vi "Teleop.vi"(10 "Match Info":T1={"Autonomous Elapsed Seconds"=0.0, "TeleOp Elapsed Seconds"=0.0, "Disabled Elapsed Seconds"=0.0, "Visited Autonomous"=FALSE, "Visited TeleOp"=FALSE, "Visited Disabled"=FALSE, "Autonomous Settings"={"Autonomous Style"=enum."Independent", "VI Refnum"=refnum}}, 11 "Call Context":T2) -> ()   [LabVIEW 2019]
doc: "This VI is called for each TeleOp packet received from the DS where the robot is not disabled. It is often used to read from the joysticks and update I/O or to update setpoints for timed control loops. It should complete and return within 20 milliseconds or it may miss DS packets."
uses:
  <vilib>/Rock Robotics/WPI/DriverStation/WPI_DriverStationDerivedRobotMode.ctl
  <vilib>/Rock Robotics/WPI/DriverStation/WPI_DriverStationMatch Info.ctl
  <vilib>/Rock Robotics/WPI/ThirdParty/JAS_Junk/TrajLib/Conv_Meters_Feet.vi
  <vilib>/Rock Robotics/WPI/ThirdParty/JAS_Junk/TrajLib/Conv_Radians_Deg.vi
  <vilib>/Rock Robotics/WPI/Utilities/WPI_GetSetVariantRefNum.vi
  <vilib>/Rock Robotics/Network Tables/NT Write Boolean Array.vi
  <vilib>/Rock Robotics/Network Tables/NT Write Numeric Array.vi
  <vilib>/Rock Robotics/WPI/Joystick/WPI_JoystickArcadeMapping.vi
  Robot Global Data.vi
  <vilib>/Rock Robotics/Network Tables/NT Read Boolean.vi
  <vilib>/Rock Robotics/Network Tables/NT Read Number.vi
  <vilib>/Rock Robotics/WPI/ThirdParty/JAS_Junk/TrajLib/Trajectory_Library.lvlib
panel:
  out "Sample Slider 0":dbl(slide) scale=0.0..5.0
  out "Sample Boolean 1":bool
  out "Sample Boolean 0":bool
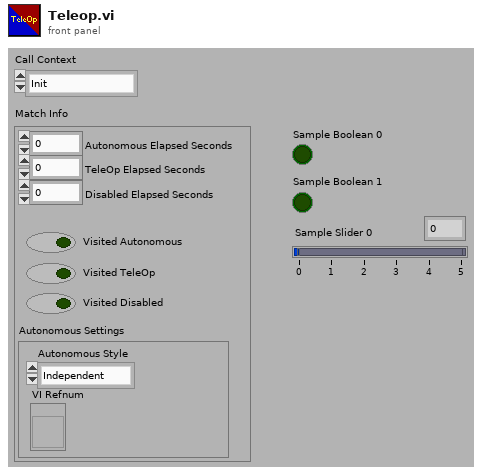
[diagram p1: front panel]
types:
  T1 = typedef "WPI_DriverStationMatch Info.ctl" = cluster{"Autonomous Elapsed Seconds":dbl, "TeleOp Elapsed Seconds":dbl, "Disabled Elapsed Seconds":dbl, "Visited Autonomous":bool, "Visited TeleOp":bool, "Visited Disabled":bool, "Autonomous Settings":cluster{"Autonomous Style":enum16{"Iterative", "Independent"}, "VI Refnum":refnum<vi>}}
  T2 = typedef "WPI_DriverStationDerivedRobotMode.ctl" = enum16{"Init", "Execute", "Stop"}
  T3 = typedef "WPI_JoystickDevRef.ctl" = cluster{"Device":T4}
  T4 = typedef "WPI_JoystickDeviceEnum.ctl" = enum16{"USB 0", "USB 1", "USB 2", "USB 3", "USB 4", "USB 5"}
  T5 = typedef "Trajectory_Library.lvlib/RAMSETE.ctl" = cluster{"B":dbl, "Zeta":dbl, "poseTolerance":T6, "poseError":T6, "Enabled":bool}
  T6 = typedef "Trajectory_Library.lvlib/POSE2D.ctl" = cluster{"TRANSLATION":T7, "ROTATION":T8}
  T7 = typedef "Trajectory_Library.lvlib/TRANSLATION2D.ctl" = cluster{"X":dbl, "Y":dbl}
  T8 = typedef "Trajectory_Library.lvlib/ROTATION2D.ctl" = cluster{"VALUE":dbl, "COS":dbl, "SIN":dbl}
  T9 = typedef "Trajectory_Library.lvlib/TRAJ_STATE.ctl" = cluster{"TimeSeconds":dbl, "Velocity":dbl, "Acceleration":dbl, "POSE":T6, "Curvature":dbl}
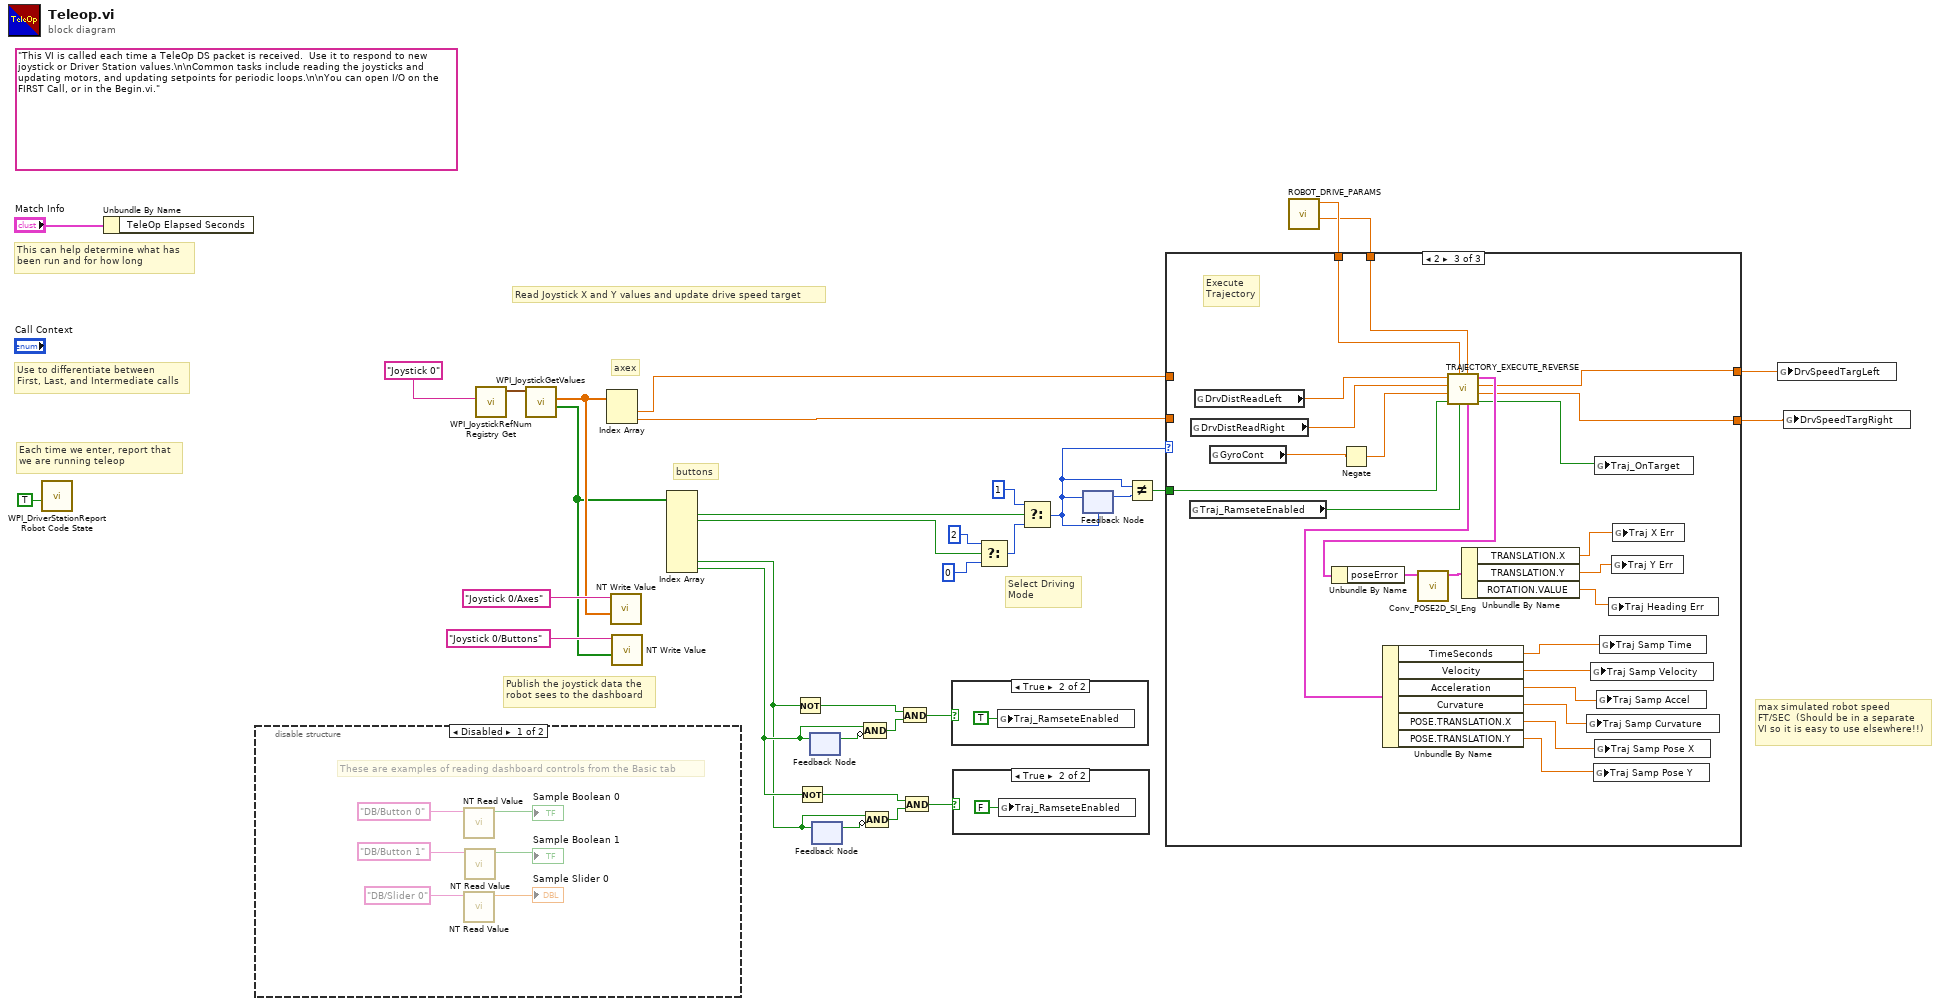
[diagram p0: block diagram]
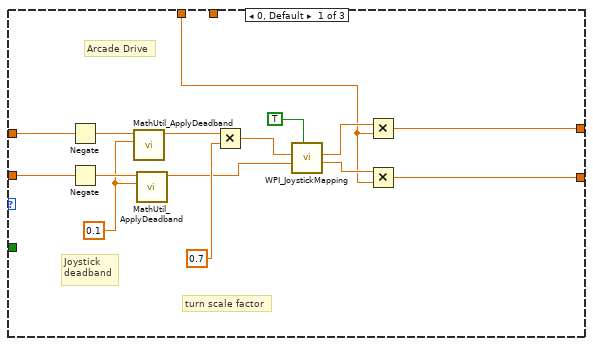
[diagram p4: hidden frame]
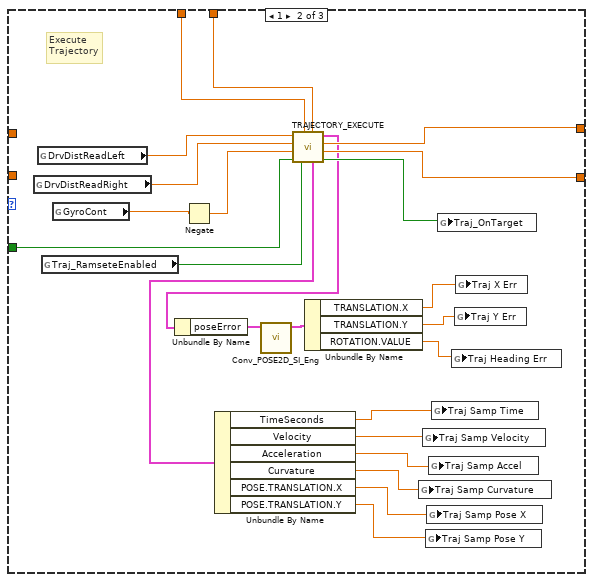
[diagram p5: hidden frame]
diagram:
  (unwired) "This VI is called each time a TeleOp DS packet is received.  Use it to respond to new joystick or Driver Station values.\n\nCommon tasks include reading the joysticks and updating motors, and updating setpoints for periodic loops.\n\nYou can open I/O on the FIRST Call, or in the Begin.vi."
  # "Select Driving\nMode"
  # "buttons"
  # "axex"
  # "max simulated robot speed\nFT/SEC  (Should be in a separate\nVI so it is easy to use elsewhere!!)"
  # "Publish the joystick data the\nrobot sees to the dashboard"
  # "Each time we enter, report that\nwe are running teleop"
  # "Use to differentiate between\nFirst, Last, and Intermediate calls"
  # "This can help determine what has\nbeen run and for how long"
  # "Read Joystick X and Y values and update drive speed target"
  n1 = call <vilib>:"WPI_DriverStationReport Robot Code State.vi"("TeleOp"=TRUE ("Autonomous")) -> ()  [unwired: 10 in, 1 out]
  n2 = Unbundle By Name("Match Info") -> ()  [unwired: 1 out]
  n3 = disable-structure shown="Disabled" {
    frame Disabled {
      # "These are examples of reading dashboard controls from the Basic tab"
      n4 = call-poly <vilib>:"NT Read Value.vi"("Name"="DB/Button 0" ("refnum name")) -> ("Boolean"=→"Sample Boolean 0":bool)  [unwired: 9 in, 1 out]
      n5 = call-poly <vilib>:"NT Read Value.vi"("Name"="DB/Slider 0" ("refnum name")) -> ("Numeric"=→"Sample Slider 0":dbl)  [unwired: 9 in, 1 out]
      n6 = call-poly <vilib>:"NT Read Value.vi"("Name"="DB/Button 1" ("refnum name")) -> ("Boolean"=→"Sample Boolean 1":bool)  [unwired: 9 in, 1 out]
    }
    frame Enabled {
    }
  }
  n7 = call <vilib>:"WPI_JoystickRefNum Registry Get.vi"("refnum name"="Joystick 0") -> ("JoystickDevRef"=w31:T3)  [unwired: 1 in, 9 out]
  n8 = call <vilib>:"WPI_JoystickGetValues.vi"("JoystickDevRef"=w31) -> ("Buttons"=w22:bool[], "Axes"=w27:dbl[])  [unwired: 6 in, 3 out]
  n9 = Index Array(array=w27) -> (element #1=w26:dbl, element #2=w25:dbl)  [unwired: 2 in]
  n10 = call-poly <vilib>:"NT Write Value.vi"("Numeric Array"=w27, "Name"="Joystick 0/Axes") -> ()  [unwired: 9 in, 1 out]
  n11 = call-poly <vilib>:"NT Write Value.vi"("Boolean Array"=w22, "Name"="Joystick 0/Buttons") -> ()  [unwired: 9 in, 1 out]
  n12 = Index Array(array=w22) -> (element #1=w20:bool, element #2=w13:bool, element #7=w1:bool, element #8=w2:bool)  [unwired: 8 in, 4 out]
  n13 = Not(x=w1) -> (.not. x?=w8:bool)
  n14 = Not(x=w2) -> (.not. x?=w5:bool)
  n15 = feedback-in #1(w2) -> ()
  n16 = feedback #1() -> (w10:bool)  [unwired: 1 in]
  n17 = feedback #2() -> (w7:bool)  [unwired: 1 in]
  n18 = feedback-in #2(w1) -> ()
  n19 = Compound Arithmetic op=AND(w2, invert w10) -> (w9:bool)
  n20 = Compound Arithmetic op=AND(w1, invert w7) -> (w6:bool)
  n21 = And(x=w8, y=w9) -> (x .and. y?=w3:bool)
  n22 = And(x=w5, y=w6) -> (x .and. y?=w4:bool)
  n23 = case shown="True" w3 {
    frame False {
    }
    frame True {
      n24 = global write "Robot Global Data.vi" "Traj_RamseteEnabled"(TRUE ("Traj_RamseteEnabled")) -> ()
    }
  }
  n25 = case shown="True" w4 {
    frame False {
    }
    frame True {
      n26 = global write "Robot Global Data.vi" "Traj_RamseteEnabled"(FALSE ("Traj_RamseteEnabled")) -> ()
    }
  }
  n27 = Select(t=2, s=w13, f=0) -> (s? t:f=w14:i32)
  n28 = Select(t=1, s=w20, f=w14) -> (s? t:f=w18:i32)
  n29 = feedback-in #3(w18) -> ()
  n30 = feedback #3(w18) -> (w19:i32)
  n31 = Not Equal?(x=w18, y=w19) -> (x != y?=w17:bool)
  n32 = call "ROBOT_DRIVE_PARAMS.vi"() -> ("Effective Wheelbase Ft"=w11:dbl, "Max Speed Ft/Sec"=w12:dbl)  [unwired: 10 in]
  n33 = case shown="2" w18 {
    tunnel: w26 -> [w55 _ _]
    tunnel: w25 -> [w54 _ _]
    tunnel: [w53 w75 w95] -> w24
    tunnel: [w52 w74 w94] -> w23
    tunnel: w17 -> [_ w80 w89]
    tunnel: w12 -> [w49 w66 w97]
    tunnel: w11 -> [_ w65 w98]
    frame 0, Default {
      w42 = 0.1 ("Deadband")
      # "Joystick\ndeadband"
      # "turn scale factor"
      # "Arcade Drive"
      n34 = Negate(x=w55) -> (-x=w44:dbl)
      n35 = Negate(x=w54) -> (-x=w43:dbl)
      n36 = call <vilib>:"MathUtil_ApplyDeadband.vi"("Deadband"=w42, "Value"=w44) -> ("Result"=w45:dbl)  [unwired: 9 in]
      n37 = call <vilib>:"MathUtil_ApplyDeadband.vi"("Deadband"=w42, "Value"=w43) -> ("Result"=w46:dbl)  [unwired: 9 in]
      n38 = Multiply(x=w45, y=0.7) -> (x*y=w47:dbl)
      n39 = call-poly <vilib>:"WPI_JoystickMapping.vi"("Square Inputs"=TRUE, "Y axis value"=w46, "X axis value"=w47) -> ("Right Motor Value"=w50:dbl, "Left Motor Value"=w51:dbl)  [unwired: 7 in]
      n40 = Multiply(x=w51, y=w49) -> (x*y=w53:dbl)
      n41 = Multiply(x=w50, y=w49) -> (x*y=w52:dbl)
    }
    frame 1 {
      # "Execute\nTrajectory"
      n42 = global read "Robot Global Data.vi" "DrvDistReadRight"() -> (w77:dbl)
      n43 = global read "Robot Global Data.vi" "DrvDistReadLeft"() -> (w78:dbl)
      n44 = global read "Robot Global Data.vi" "Traj_RamseteEnabled"() -> (w57:bool)
      n45 = global read "Robot Global Data.vi" "GyroCont"() -> (w79:dbl)
      n46 = Negate(x=w79) -> (-x=w76:dbl)
      n47 = call "TRAJECTORY_EXECUTE.vi"("Track Width FT"=w65, "RamseteEnable"=w57, "Max Speed\nFT/SEC"=w66, "Init"=w80, "Gyro Continous\n (inc counterclockwise)"=w76, "Right Distance"=w77, "Left Distance"=w78) -> ("AtReference"=w73:bool, "Right Speed Target"=w74:dbl, "Left Speed Target"=w75:dbl, "outRAMSETE (SI)"=w72:T5, "OutputTRAJ_STATE (SI)"=w58:T9)
      n48 = Unbundle By Name(w72) -> ("poseError"=w71:T6)
      n49 = Unbundle By Name(w58) -> ("TimeSeconds"=w64:dbl, "Velocity"=w63:dbl, "Acceleration"=w62:dbl, "Curvature"=w61:dbl, "POSE.TRANSLATION.X"=w60:dbl, "POSE.TRANSLATION.Y"=w59:dbl)
      n50 = call <vilib>:"Conv_POSE2D_SI_Eng.vi"("Err Pose in SI"=w71) -> ("Err Pose out ENG"=w70:T6)  [unwired: 10 in]
      n51 = Unbundle By Name(w70) -> ("TRANSLATION.X"=w69:dbl, "TRANSLATION.Y"=w68:dbl, "ROTATION.VALUE"=w67:dbl)
      n52 = global write "Robot Global Data.vi" "Traj Samp Curvature"(w61) -> ()
      n53 = global write "Robot Global Data.vi" "Traj Samp Velocity"(w63) -> ()
      n54 = global write "Robot Global Data.vi" "Traj Samp Pose Y"(w59) -> ()
      n55 = global write "Robot Global Data.vi" "Traj Samp Pose X"(w60) -> ()
      n56 = global write "Robot Global Data.vi" "Traj Samp Accel"(w62) -> ()
      n57 = global write "Robot Global Data.vi" "Traj Samp Time"(w64) -> ()
      n58 = global write "Robot Global Data.vi" "Traj_OnTarget"(w73) -> ()
      n59 = global write "Robot Global Data.vi" "Traj Heading Err"(w67) -> ()
      n60 = global write "Robot Global Data.vi" "Traj Y Err"(w68) -> ()
      n61 = global write "Robot Global Data.vi" "Traj X Err"(w69) -> ()
    }
    frame 2 {
      # "Execute\nTrajectory"
      n62 = global read "Robot Global Data.vi" "Traj_RamseteEnabled"() -> (w81:bool)
      n63 = global read "Robot Global Data.vi" "DrvDistReadRight"() -> (w91:dbl)
      n64 = global read "Robot Global Data.vi" "DrvDistReadLeft"() -> (w92:dbl)
      n65 = global read "Robot Global Data.vi" "GyroCont"() -> (w104:dbl)
      n66 = Negate(x=w104) -> (-x=w90:dbl)
      n67 = call "TRAJECTORY_EXECUTE_REVERSE.vi"("Track Width FT"=w98, "RamseteEnable"=w81, "Max Speed\nFT/SEC"=w97, "Init"=w89, "Gyro Continous\n (inc counterclockwise)"=w90, "Right Distance"=w91, "Left Distance"=w92) -> ("AtReference"=w93:bool, "Right Speed Target"=w94:dbl, "Left Speed Target"=w95:dbl, "outRAMSETE (SI)"=w96:T5, "OutputTRAJ_STATE (SI)"=w82:T9)
      n68 = Unbundle By Name(w96) -> ("poseError"=w103:T6)
      n69 = Unbundle By Name(w82) -> ("TimeSeconds"=w88:dbl, "Velocity"=w87:dbl, "Acceleration"=w86:dbl, "Curvature"=w85:dbl, "POSE.TRANSLATION.X"=w84:dbl, "POSE.TRANSLATION.Y"=w83:dbl)
      n70 = call <vilib>:"Conv_POSE2D_SI_Eng.vi"("Err Pose in SI"=w103) -> ("Err Pose out ENG"=w102:T6)  [unwired: 10 in]
      n71 = Unbundle By Name(w102) -> ("TRANSLATION.X"=w101:dbl, "TRANSLATION.Y"=w100:dbl, "ROTATION.VALUE"=w99:dbl)
      n72 = global write "Robot Global Data.vi" "Traj Samp Curvature"(w85) -> ()
      n73 = global write "Robot Global Data.vi" "Traj Samp Velocity"(w87) -> ()
      n74 = global write "Robot Global Data.vi" "Traj Samp Pose Y"(w83) -> ()
      n75 = global write "Robot Global Data.vi" "Traj_OnTarget"(w93) -> ()
      n76 = global write "Robot Global Data.vi" "Traj Samp Pose X"(w84) -> ()
      n77 = global write "Robot Global Data.vi" "Traj Samp Accel"(w86) -> ()
      n78 = global write "Robot Global Data.vi" "Traj Samp Time"(w88) -> ()
      n79 = global write "Robot Global Data.vi" "Traj Heading Err"(w99) -> ()
      n80 = global write "Robot Global Data.vi" "Traj Y Err"(w100) -> ()
      n81 = global write "Robot Global Data.vi" "Traj X Err"(w101) -> ()
    }
  }
  n82 = global write "Robot Global Data.vi" "DrvSpeedTargLeft"(w24) -> ()
  n83 = global write "Robot Global Data.vi" "DrvSpeedTargRight"(w23) -> ()
